vi "INIT arms.vi"(8 "error in (no error)":errorcluster) -> (0 "error out":errorcluster)   [LabVIEW 2023]
uses:
  Global INIT.vi
  <vilib>/Rock Robotics/WPI/ThirdParty/REV Robotics/REVLib/Typedef/Spark MAX Limit Direction.ctl
  <vilib>/Rock Robotics/WPI/ThirdParty/REV Robotics/REVLib/SubVI/Public/SPARK Configure Soft Limit Forward.vi
  <vilib>/Rock Robotics/WPI/ThirdParty/REV Robotics/REVLib/SubVI/Public/SPARK Configure Soft Limit Reverse.vi
panel:
  out "set soft\nlimit max (revs)":dbl
  in  "%max limit":i16=95 min=50 max=100 step=1
  out "sprocket\nC (in/rev)":dbl
  out "shaft revs\nto max extension":dbl
  out "sprocket revs\nto max extension":dbl
  in  "gear ratio\n(driven/driver)\nshaft to sprocket":dbl=1.0 format="%_5f"
  in  "sprocket\npitch diameter (in)":dbl=1.123 format="%_5f"
  in  "max arm\nextension (in)":dbl=21.87 format="%_5f"
  # "SOFT LIMITS for arms:\n   Mechanism uses NEO motor on 16:1 planetary Sports gearbox driving a \n25-series 14-tooth sprocket on a 1/2\" hex output shaft.\n\nvertical rise of the arm = revs of circumference of sprocket pitch-diameter\n\nmotor kPositionCoefficient already takes the 16:1 into account so Get POS should give the planetary shaft position.  An extra gear ratio is included in case of a gear train after shaft."
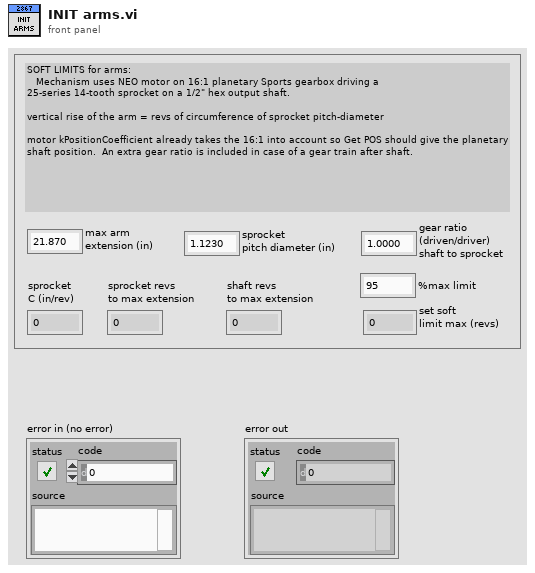
[diagram p1: front panel]
types:
  T1 = typedef "ctrl arm motor.ctl" = cluster{" motor":T2, "limit polarities":T8}
  T2 = typedef "ctrl swerve motor.ctl" = cluster{"description":string, "MOTOR SELECT":T3, "Installed?":bool, "CAN ID":u8, "refnum name":string, "Invert":bool, "Idle Mode":T4, "Current limiting":T5, "MOTOR PIDF coefficients":T6, "gear ratio":dbl}
  T3 = typedef "ctrl MOTOR SELECT.ctl" = i16
  T4 = typedef "Spark MAX Idle Mode.ctl" = enum16{"Coast", "Brake"}
  T5 = typedef "ctrl Spark MAX current limiting.ctl" = cluster{"Linearized":bool, "Free Speed (A)":dbl, "Primay (A)":dbl, "Limit RPM (0)":u32}
  T6 = typedef "ctrl motor PIDF coefficients.ctl" = cluster{"PIDF":cluster{"P Gain":dbl, "I Gain":dbl, "D Gain":dbl, "F Gain":dbl, "I Zone":dbl, "Min Output":dbl, "Max Output":dbl}, "Smart Motion":T7}
  T7 = typedef "Spark MAX Smart Motion Parameters.ctl" = cluster{"Max Velocity":dbl, "Max Acceleration":dbl, "Minimum Velocity Output":dbl, "Allowed Closed Loop Error":dbl}
  T8 = typedef "ctrl limit polarity.ctl" = cluster{"Forward limit":T9, "Reverse limit":T9}
  T9 = typedef "Spark MAX Limit Switch Polarity.ctl" = enum16{"Normally Open", "Normally Closed"}
  T10 = typedef "Spark MAX Limit Direction.ctl" = enum16{"Forward Limit", "Reverse Limit"}
  T11 = typedef "WPI_MotorControlDeviceRef.ctl" = cluster{"DeviceStatus":errorcluster, "Type":T12, "PWM":cluster{"PWM Channel":T13, "DeadBand":T14}, "CAN":cluster{"Device Number":u8, "SetOutput VI Ref":variant, "GetOutput VI Ref":variant, "Enable VI Ref":variant, "Disable VI Ref":variant, "Data":variant}, "Invert":bool, "DIO PWM":cluster{"PWM \"Enable\" Channel":T13, "DIOChannel":T15, "PWM Rate":dbl}}
  T12 = typedef "WPI_MotorControlType.ctl" = enum16{"PWM", "CAN", "DIO PWM"}
  T13 = typedef "FPGA_DIOPWMChannel.ctl" = enum8{"PWM 0", "PWM 1", "PWM 2", "PWM 3", "PWM 4", "PWM 5", "PWM 6", "PWM 7", "PWM 8", "PWM 9", "PWM MXP 0", "PWM MXP 1", "PWM MXP 2", "PWM MXP 3", "PWM MXP 4", "PWM MXP 5", "PWM MXP 6", "PWM MXP 7", "PWM MXP 8", "PWM MXP 9", "Invalid"}
  T14 = typedef "WPI_PWMDeadband.ctl" = cluster{"Name":string, "maxPositivePwm":i32, "minPositivePwm":i32, "centerPwm":i32, "maxNegativePwm":i32, "minNegativePwm":i32, "angularRange":u16}
  T15 = typedef "FPGA_DIOChannel.ctl" = enum8{"DIO 0", "DIO 1", "DIO 2", "DIO 3", "DIO 4", "DIO 5", "DIO 6", "DIO 7", "DIO 8", "DIO 9", "DIO MXP 0", "DIO MXP 1", "DIO MXP 2", "DIO MXP 3", "DIO MXP 4", "DIO MXP 5", "DIO MXP 6", "DIO MXP 7", "DIO MXP 8", "DIO MXP 9", "DIO MXP 10", "DIO MXP 11", "DIO MXP 12", "DIO MXP 13", "DIO MXP 14", "DIO MXP 15", "SPI Port CS1", "SPI Port CS2", "SPI Port CS3", "SPI Port MISO", "SPI Port MOSI", "Invalid"}
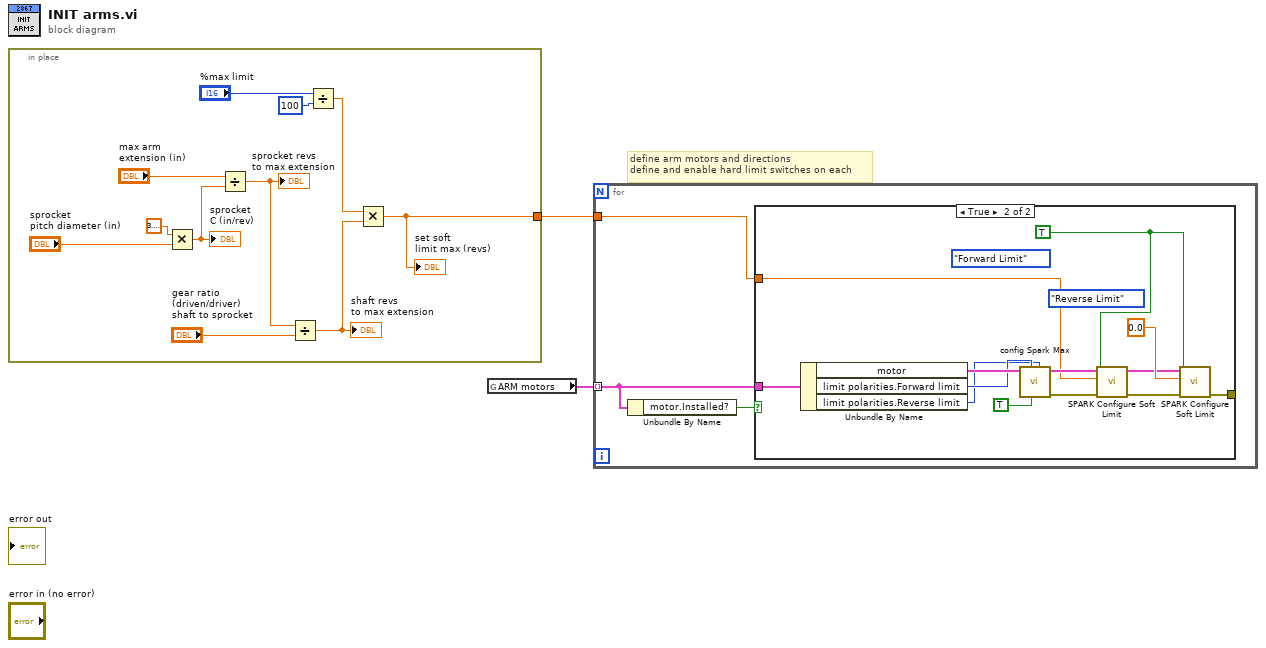
[diagram p0: block diagram]
diagram:
  # "define arm motors and directions\ndefine and enable hard limit switches on each"
  n1 = in-place {
    in-place-border: [w3] -> w1
    n2 = Multiply(x=3.141592653589793, y="sprocket\npitch diameter (in)") -> (x*y=w11:dbl)
    "sprocket\nC (in/rev)" <- w11
    n3 = Divide(x="max arm\nextension (in)", y=w11) -> (x/y=w9:dbl)
    "sprocket revs\nto max extension" <- w9
    n4 = Divide(x=w9, y="gear ratio\n(driven/driver)\nshaft to sprocket") -> (x/y=w4:dbl)
    "shaft revs\nto max extension" <- w4
    n5 = Divide(x="%max limit", y=i16 100) -> (x/y=w5:dbl)
    n6 = Multiply(x=w5, y=w4) -> (x*y=w3:dbl)
    "set soft\nlimit max (revs)" <- w3
  }
  n7 = global read "Global INIT.vi" "ARM motors"() -> (w2:T1[])
  n8 = for {
    tunnel: w2 -> [w15] mode=indexing
    tunnel: w1 -> [w14]
    n9 = Unbundle By Name(w15) -> ("motor.Installed?"=w16:bool)
    n10 = case shown="True" w16 {
      tunnel: w15 -> [_ w28]
      tunnel: [_ w19] -> _
      tunnel: w14 -> [_ w17]
      frame False {
      }
      frame True {
        (unwired) Spark_MAX_Limit_Direction."Reverse Limit" ("Soft Limit Switch")
        w18 = TRUE ("Enabled? (T)")
        (unwired) Spark_MAX_Limit_Direction."Forward Limit" ("Soft Limit Switch")
        n11 = Unbundle By Name(w28) -> ("motor"=w29:T2, "limit polarities.Forward limit"=w27:T9, "limit polarities.Reverse limit"=w26:T9)
        n12 = call "config Spark Max.vi"("Reverse Limit switch"=w26, "LIMIT SW\nEnabled?"=TRUE ("LIMIT SW\nEnabled?"), "Forward Limit switch"=w27, "motor\ndefaults"=w29) -> ("error out"=w22:errorcluster, "MotorControlDevRef"=w21:T11)  [unwired: 6 in]
        n13 = call-poly <vilib>:"SPARK Configure Soft Limit.vi"("error in"=w22, "Enabled? (T)"=w18, "Soft Limit"=w17, "MotorControlDeviceRef in"=w21) -> ("error out"=w24:errorcluster, "MotorControlDeviceRef out"=w20:T11)  [unwired: 6 in]
        n14 = call-poly <vilib>:"SPARK Configure Soft Limit.vi"("error in"=w24, "Enabled? (T)"=w18, "Soft Limit"=0.0 ("Soft Limit (0)"), "MotorControlDeviceRef in"=w20) -> ("error out"=w19:errorcluster)  [unwired: 6 in, 1 out]
      }
    }
  }
